vi "Set_table_heads.vi"(4 "additional row width":i16, 5 "Columm additional width":i16, 8 "error in (no error)":errorcluster, 9 "Row texts":string[](array[string]), 10 "Column texts":string[](array[string]), 11 "Table ref in":refnum<vi>) -> (0 "error out":errorcluster, 3 "Table ref out":refnum<vi>)   [LabVIEW 2016]
uses:
  <vilib>/Utility/miscctls.llb/LVRowAndColumnTypeDef.ctl
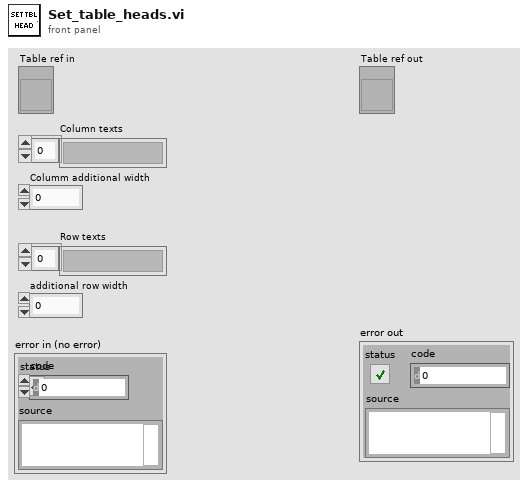
[diagram p1: front panel]
types:
  T1 = typedef "LVRowAndColumnTypeDef.ctl" = cluster{"Row":i32, "Column":i32}
  T2 = cluster{"Font Name:":string, "Size":i16, "Strikeout?":bool, "Italic?":bool, "Underline?":bool, "Outline?":bool, "Shadow?":bool, "Bold?":bool}
  T3 = typedef "LVFontTypeDef.ctl" = cluster{"Font Name":string, "Size":u16, "Bold":bool, "Italic":bool, "Underline":bool, "Strikeout":bool, "Color":u32}
  T4 = cluster{"left":i16, "top":i16, "right":i16, "bottom":i16}
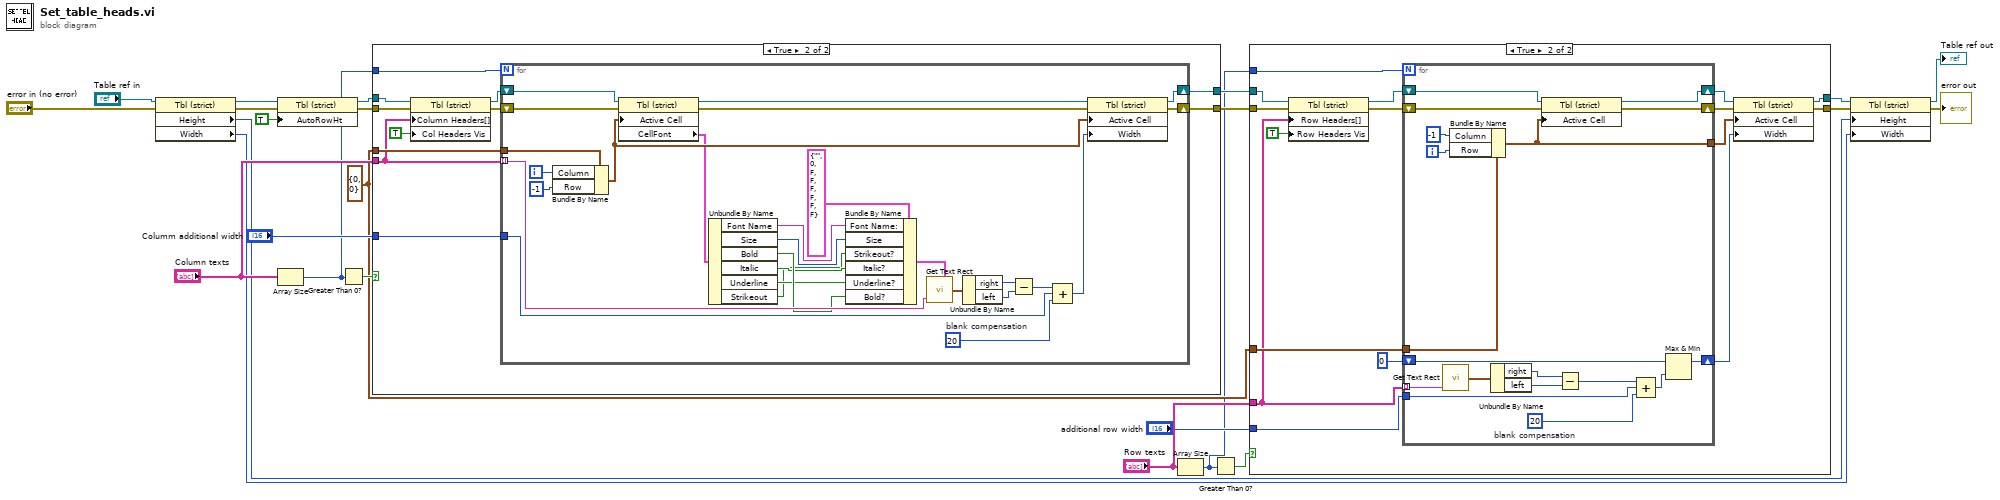
[diagram p0: block diagram]
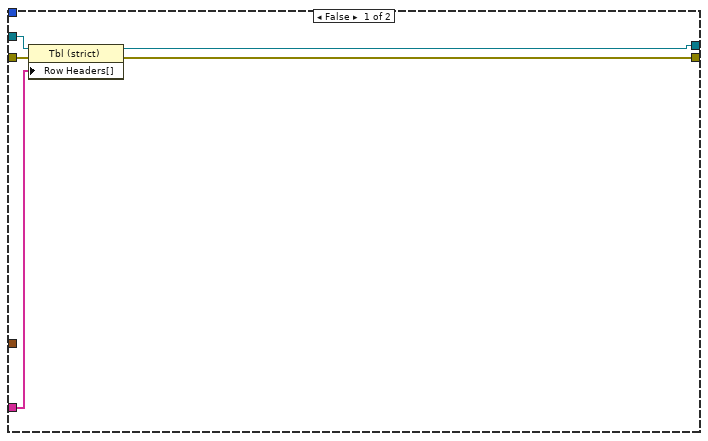
[diagram p2: hidden frame]
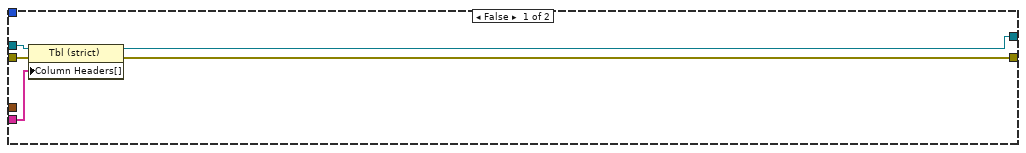
[diagram p3: hidden frame]
diagram:
  w20 = T1 {"Row"=0, "Column"=0} ("Active Cell:Active Cell")
  n1 = property on="Property Node" class="Tbl (strict)"(reference="Table ref in", error in="error in (no error)") -> (reference out=w12:refnum<vi>, error out=w11:errorcluster, "Height"=w6:u32, "Width"=w5:u32)
  n2 = property on="Property Node" class="Tbl (strict)"(reference=w12, error in=w11, "AutoRowHt"=TRUE ("Autosizing Row Height")) -> (reference out=w17:refnum<vi>, error out=w18:errorcluster)
  n3 = Array Size(array="Column texts") -> (size(s)=w2:i32)
  n4 = Greater Than 0?(x=w2) -> (x > 0?=w23:bool)
  n5 = case shown="True" w23 {
    tunnel: "Columm additional width" -> [_ w40]
    tunnel: w20 -> [_ w39]
    tunnel: "Column texts" -> [w29 w36]
    tunnel: w17 -> [w28 w38]
    tunnel: w18 -> [w27 w37]
    tunnel: [w26 w32] -> w4
    tunnel: [w25 w31] -> w3
    tunnel: w2 -> [_ w30]
    frame False {
      n6 = property on="Property Node" class="Tbl (strict)"(reference=w28, error in=w27, "Column Headers[]"=w29) -> (reference out=w26:refnum<vi>, error out=w25:errorcluster)
    }
    frame True {
      n7 = property on="Property Node" class="Tbl (strict)"(reference=w38, error in=w37, "Column Headers[]"=w36, "Col Headers Vis"=TRUE ("Visible Items:Column Headers Visible")) -> (reference out=w34:refnum<vi>, error out=w33:errorcluster)
      n8 = for {
        N: w30 -> [_]
        tunnel: w36 -> [w63] mode=indexing
        tunnel: w40 -> [w62]
        tunnel: w39 -> [w61]
        shift-right: [w58] -> w31
        shift-left: w33 -> [w52]
        shift-right: [w57] -> w32
        shift-left: w34 -> [w54]
        i -> [w60]
        w55 = i16 20  # blank compensation
        n9 = Bundle By Name(cluster=w61, "Column"=w60, "Row"=-1) -> (w53:T1)
        n10 = property on="Property Node" class="Tbl (strict)"(reference=w54, error in=w52, "Active Cell"=w53) -> (reference out=w50:refnum<vi>, error out=w51:errorcluster, "CellFont"=w48:T3)
        n11 = Unbundle By Name(w48) -> ("Font Name"=w47:string, "Size"=w46:u16, "Bold"=w45:bool, "Italic"=w44:bool, "Underline"=w43:bool, "Strikeout"=w42:bool)
        n12 = Bundle By Name(cluster=T2 {"Font Name:"="", "Size"=0, "Strikeout?"=FALSE, "Italic?"=FALSE, "Underline?"=FALSE, "Outline?"=FALSE, "Shadow?"=FALSE, "Bold?"=FALSE} ("[user-specified font]"), "Font Name:"=w47, "Size"=w46, "Strikeout?"=w42, "Italic?"=w44, "Underline?"=w43, "Bold?"=w45) -> (w41:T2)
        n13 = call <vilib>:"Get Text Rect.vi"("text"=w63, "[user-specified font]"=w41) -> ("rect"=w64:T4)  [unwired: 7 in]
        n14 = Unbundle By Name(w64) -> ("right"=w65:i16, "left"=w66:i16)
        n15 = Subtract(x=w65, y=w66) -> (x-y=w67:i16)
        n16 = Compound Arithmetic op=ADD(w67, w62, w55) -> (w59:i16)
        n17 = property on="Property Node" class="Tbl (strict)"(reference=w50, error in=w51, "Active Cell"=w53, "Width"=w59) -> (reference out=w57:refnum<vi>, error out=w58:errorcluster)
      }
    }
  }
  n18 = Array Size(array="Row texts") -> (size(s)=w1:i32)
  n19 = Greater Than 0?(x=w1) -> (x > 0?=w21:bool)
  n20 = case shown="True" w21 {
    tunnel: w20 -> [_ w88]
    tunnel: "Row texts" -> [w68 w85]
    tunnel: w4 -> [w72 w87]
    tunnel: w3 -> [w70 w86]
    tunnel: [w71 w77] -> w10
    tunnel: [w69 w75] -> w9
    tunnel: w1 -> [_ w81]
    tunnel: "additional row width" -> [_ w80]
    frame False {
      n21 = property on="Property Node" class="Tbl (strict)"(reference=w72, error in=w70, "Row Headers[]"=w68) -> (reference out=w71:refnum<vi>, error out=w69:errorcluster)
    }
    frame True {
      n22 = property on="Property Node" class="Tbl (strict)"(reference=w87, error in=w86, "Row Headers[]"=w85, "Row Headers Vis"=TRUE ("Visible Items:Column Headers Visible")) -> (reference out=w83:refnum<vi>, error out=w82:errorcluster)
      n23 = for {
        N: w81 -> [_]
        tunnel: w85 -> [w102] mode=indexing
        tunnel: w88 -> [w101]
        shift-right: [w97] -> w76
        shift-left: w82 -> [w98]
        shift-right: [w96] -> w78
        shift-left: w83 -> [w99]
        tunnel: w80 -> [w95]
        shift-right: [w90] -> w73
        shift-left: i16 0 -> [w91]
        tunnel: [w89] -> w74
        i -> [w100]
        w93 = i16 20  # blank compensation
        n24 = call <vilib>:"Get Text Rect.vi"("text"=w102) -> ("rect"=w103:T4)  [unwired: 8 in]
        n25 = Bundle By Name(cluster=w101, "Column"=-1, "Row"=w100) -> (w89:T1)
        n26 = Unbundle By Name(w103) -> ("right"=w104:i16, "left"=w105:i16)
        n27 = property on="Property Node" class="Tbl (strict)"(reference=w99, error in=w98, "Active Cell"=w89) -> (reference out=w96:refnum<vi>, error out=w97:errorcluster)
        n28 = Subtract(x=w104, y=w105) -> (x-y=w106:i16)
        n29 = Compound Arithmetic op=ADD(w106, w95, w93) -> (w92:i16)
        n30 = Max & Min(x=w91, y=w92) -> (max(x,y)=w90:i16)  [unwired: 1 out]
      }
      n31 = property on="Property Node" class="Tbl (strict)"(reference=w78, error in=w76, "Active Cell"=w74, "Width"=w73) -> (reference out=w77:refnum<vi>, error out=w75:errorcluster)
    }
  }
  n32 = property on="Property Node" class="Tbl (strict)"(reference=w10, error in=w9, "Height"=w6, "Width"=w5) -> (reference out=→"Table ref out":refnum<vi>, error out=→"error out":errorcluster)
